vi "欧姆龙PLC通讯Fans UDP-读PLC寄存器.vi"(0 "UDP网络连接输入":refnum<k16>, 5 "IP":u32, 7 "端口Port":u16, 9 "读PLC寄存器编码字符串":string, 11 "错误输入（无错误）":errorcluster) -> (4 "UDP网络连接输出":refnum<k16>, 10 "data out":string, 15 "错误输出":errorcluster)   [LabVIEW 2014]
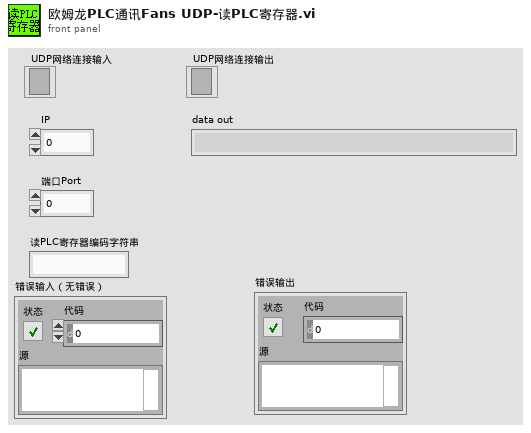
[diagram p1: front panel]
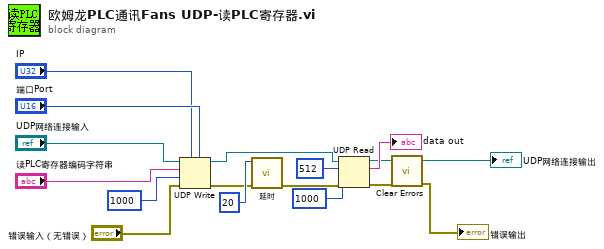
[diagram p0: block diagram]
diagram:
  n1 = UDP Write(address="IP", port or service name="端口Port", connection ID="UDP网络连接输入", data in="读PLC寄存器编码字符串", 8:"错误输入（无错误）", 9:1000 ("超时毫秒(25000)")) -> (error out=w8:errorcluster, 3:w9:refnum<k16>)
  n2 = call "延时.vi"("错误in"=w8, "等待时间（毫秒）"=u32 20) -> ("错误in"=w10:errorcluster)  [unwired: 9 in]
  n3 = UDP Read(connection ID=w9, max size (548)=512 ("读取的字节"), timeout ms (25000)=1000 ("超时毫秒(25000)"), 8:w10) -> (data out=→"data out":string, error out=w3:errorcluster, 3:→"UDP网络连接输出":refnum<k16>)  [unwired: 2 out]
  n4 = call <vilib>:"Clear Errors.vi"("error in (no error)"=w3) -> ("error out"=→"错误输出":errorcluster)  [unwired: 5 in, 1 out]
